vi "backup_strain_test_v4.vi"() -> ()   [LabVIEW 2014]
uses:
  <vilib>/LabVIEW Targets/FPGA/cRIO/shared/nicrio_ModuleControls/nicrio_cRIO-9237_DataRatesRing.ctl
  <vilib>/LabVIEW Targets/FPGA/cRIO/shared/nicrio_ModuleControls/nicrio_cRIO-9237_ExcitationVoltageRing.ctl
  <vilib>/rvi/Emulation/niFpgaGetClockAttributes.vi
  <vilib>/rvi/Emulation/niFpgaSctlEmulationGetInTimedLoop.vi
  <vilib>/rvi/Emulation/niFpgaEmulationReportErrorSimple.vi
  <vilib>/rvi/Emulation/niFpgaProcessEmulError.vi
  <vilib>/rvi/interface/RandomDataEmulation/nirviRandomDataMultiElementFPGAFIFO.vi
  <instcachedir>/0/nirviRandomDataMultiElementFPGAFIFO_AD0CFC12EF974623A9C2E4184BC062B2.lvgen/nirviRandomDataMultiElementFPGAFIFO_AD0CFC12EF974623A9C2E4184BC062B2_023.vi
  <vilib>/rvi/interface/RandomDataEmulation/niFpgaRandomDataHandleErrors.vi
  <vilib>/rvi/Emulation/niFpgaCriticalErrorInLSC.vi
  <vilib>/rvi/eio/common/nirviEmuTemplatePropertySet_errors.vi
  <vilib>/rvi/eio/common/nirviEmuTemplateMethod_errors.vi
  <vilib>/rvi/DataTransferAndStorage/Container/XNode/niFpgaContainer.xnode
  <vilib>/rvi/interface/RandomDataEmulation/nirviRandomDataFpgaMultiElementTemplate.vi
  <vilib>/eio/EIOPropertyNode/EIOPropertyNode.xnode
  <vilib>/eio/EIONode/EIONode.xnode
  <vilib>/rvi/Analysis/measure/butterworth/XNode/niFpgaButterworthFilter.xnode
  <vilib>/rvi/eio/common/nirviEmuTemplatePropertyGet_errors.vi
  <vilib>/rvi/eio/common/nirviEmuTemplatePropertyGet_noerrors.vi
  <vilib>/rvi/eio/common/nirviEmuTemplatePropertySet_noerrors.vi
panel:
  out "Strain(mean)":fxp<+/-,32,4>
  out "Loop rate (kHz)":fxp<+/-,36,7>
  in  "Strain filter coeff.":i32[](array[numeric])=[-850883994, 1909449570, 3794062, -975456236, 2033039520, 4039635]
  out "Force":fxp<+/-,32,10>
  out "Strain":fxp<+/-,42,8>
  out "Fileterd data":fxp<+/-,32,4>
  out "Raw Force":fxp<+/-,32,10>
  in  "S/F coeff":fxp<+/-,41,4>
  out "Raw Strain":fxp<+/-,42,8>
  in  "Reset":bool
  in  "Stop":bool
  out "Mod6/AI2":fxp<+/-,32,4>
  in  "Shunt Cal Enable":bool
  in  "Half-Bridge Enable":bool
  in  "Excitation Voltage":T1 items=["2.5 Volts", "3.3 Volts", "5.0 Volts", "10.0 Volts", "External Excitation"]
  in  "Data Rate":T2=1 items=["50.000 kS/s (NI 9237)"=1, "25.000 kS/s (NI 9237)"=2, "16.667 kS/s (NI 9237)"=3, "12.500 kS/s (NI 9237)"=4, "10.000 kS/s (NI 9237)"=5, "8.333 kS/s (NI 9237)"=6, "7.143 kS/s (NI 9237)"=7, "6.250 kS/s (NI 9237)"=8, "5.556 kS/s (NI 9237)"=9, "5.000 kS/s (NI 9237)"=10, "4.545 kS/s (NI 9237)"=11, "4.167 kS/s (NI 9237)"=12, "3.846 kS/s (NI 9237)"=13, "3.571 kS/s (NI 9237)"=14, "3.333 kS/s (NI 9237)"=15, "3.125 kS/s (NI 9237)"=16, "2.941 kS/s (NI 9237)"=17, "2.778 kS/s (NI 9237)"=18, "2.632 kS/s (NI 9237)"=19, "2.500 kS/s (NI 9237)"=20, "2.381 kS/s (NI 9237)"=21, "2.273 kS/s (NI 9237)"=22, "2.174 kS/s (NI 9237)"=23, "2.083 kS/s (NI 9237)"=24, "2.000 kS/s (NI 9237)"=25, "1.923 kS/s (NI 9237)"=26, "1.852 kS/s (NI 9237)"=27, "1.786 kS/s (NI 9237)"=28, "1.724 kS/s (NI 9237)"=29, "1.667 kS/s (NI 9237)"=30, "1.613 kS/s (NI 9237)"=31]
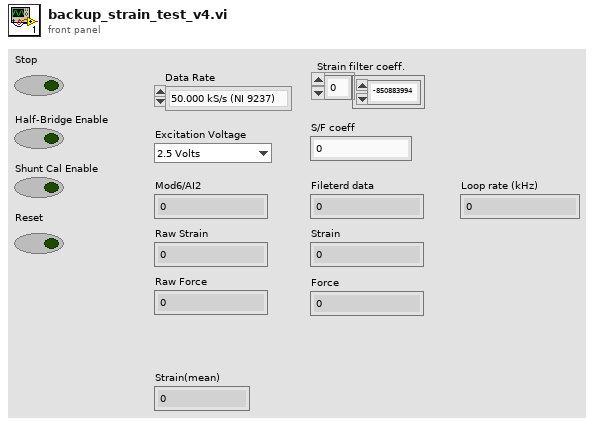
[diagram p1: front panel]
types:
  T1 = typedef "nicrio_cRIO-9237_ExcitationVoltageRing.ctl" = u8
  T2 = typedef "nicrio_cRIO-9237_DataRatesRing.ctl" = u8
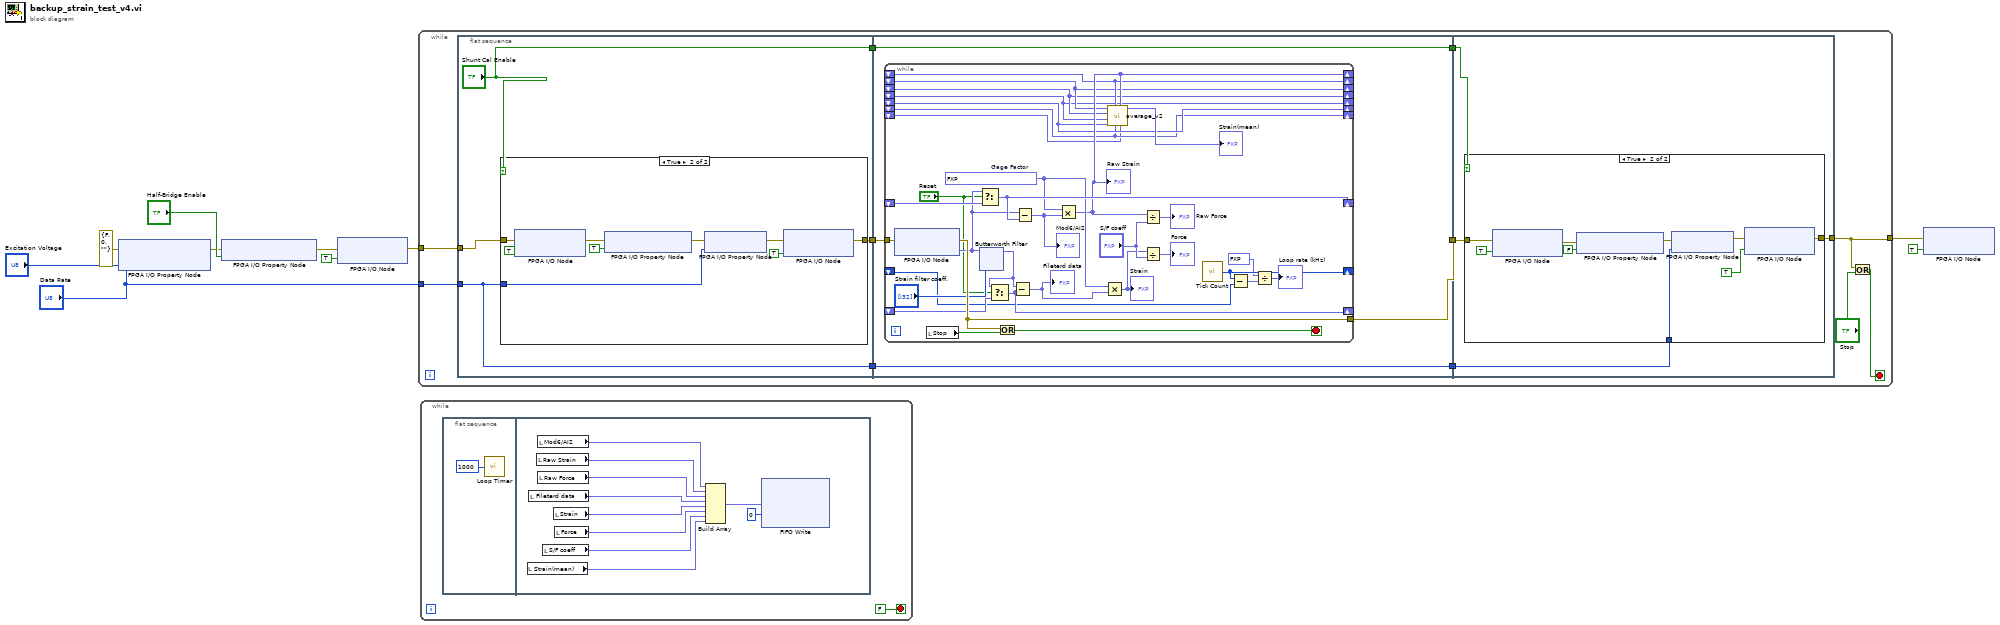
[diagram p0: block diagram]
diagram:
  n1 = xnode "FPGA I/O Property Node"("error in"=errorcluster {"status"=FALSE, "code"=0, "source"=""}, "Data Rate"="Data Rate", "Excitation Voltage"="Excitation Voltage") -> ("error out"=w7:errorcluster)  [unwired: 1 in, 1 out]
  n2 = xnode "FPGA I/O Property Node"("error in"=w7, "Half-Bridge Enable"="Half-Bridge Enable") -> ("error out"=w6:errorcluster)  [unwired: 1 in, 1 out]
  n3 = xnode "FPGA I/O Node"("error in"=w6, "Mod6/Start"=TRUE) -> ("error out"=w4:errorcluster)  [unwired: 1 in, 1 out]
  n4 = while {
    tunnel: w4 -> [w21]
    tunnel: "Data Rate" -> [w20]
    tunnel: [w12] -> w2
    stop <- w13 stop-if-true
    n5 = flat-sequence {
      tunnel: w21 -> [w25]
      tunnel: w20 -> [w24]
      tunnel: [w24] -> w19
      tunnel: ["Shunt Cal Enable"] -> w18
      tunnel: [w22] -> w17
      tunnel: w19 -> [w37]
      tunnel: w18 -> [w38]
      tunnel: w17 -> [w39]
      tunnel: [w38] -> w16
      tunnel: [w36] -> w15
      tunnel: [w37] -> w14
      tunnel: w16 -> [w84]
      tunnel: w15 -> [w83]
      tunnel: w14 -> [w82]
      tunnel: [w81] -> w12
      frame #0 {
        n6 = case shown="True" "Shunt Cal Enable" {
          tunnel: w25 -> [w26 w33]
          tunnel: w24 -> [_ w31]
          tunnel: [w26 w28] -> w22
          frame False {
          }
          frame True {
            n7 = xnode "FPGA I/O Node"("error in"=w33, "Mod6/Stop"=TRUE) -> ("error out"=w34:errorcluster)  [unwired: 1 in, 1 out]
            n8 = xnode "FPGA I/O Property Node"("error in"=w34, "Shunt Cal Enable"=TRUE) -> ("error out"=w32:errorcluster)  [unwired: 1 in, 1 out]
            n9 = xnode "FPGA I/O Property Node"("error in"=w32, "Data Rate"=w31) -> ("error out"=w30:errorcluster)  [unwired: 1 in, 1 out]
            n10 = xnode "FPGA I/O Node"("error in"=w30, "Mod6/Start"=TRUE) -> ("error out"=w28:errorcluster)  [unwired: 1 in, 1 out]
          }
        }
      }
      frame #1 {
        n11 = while {
          tunnel: w39 -> [w72]
          tunnel: [w70] -> w36
          shift-right: [w68] -> _
          shift-left: _ -> [w69]
          shift-right: [w64] -> _
          shift-left: _ -> [w65]
          shift-right: [w53] -> _
          shift-left: _ -> [w54]
          shift-right: [w48] -> _
          shift-left: _ -> [w46]
          shift-right: [w46] -> _
          shift-left: _ -> [w45]
          shift-right: [w45] -> _
          shift-left: _ -> [w44]
          shift-right: [w44] -> _
          shift-left: _ -> [w43]
          shift-right: [w43] -> _
          shift-left: _ -> [w42]
          shift-right: [w42] -> _
          shift-left: _ -> [w41]
          shift-right: [w41] -> _
          shift-left: _ -> [w40]
          stop <- w57 stop-if-true
          w62 = fxp<+,20,2> 2.115001678466797  # Gage Factor
          n12 = xnode "FPGA I/O Node"("error in"=w72) -> ("error out"=w70:errorcluster, "Mod6/AI2"=w66:fxp<+/-,24,-4>)  [unwired: 1 in, 1 out]
          n13 = local read "Stop"() -> (w71:bool)
          n14 = xnode "Butterworth Filter"("input data"=w66, "scaled coefficients"="Strain filter coeff.") -> ("output data"=w63:fxp<+/-,28,0>)  [unwired: 1 in]
          n15 = Select(t=w66, s="Reset", f=w69) -> (s? t:f=w68:fxp<+/-,24,-4>)
          n16 = Select(t=w63, s="Reset", f=w65) -> (s? t:f=w64:fxp<+/-,28,0>)
          n17 = Or(x=w70, y=w71) -> (x .or. y?=w57:bool)
          n18 = Subtract(x=w63, y=w64) -> (x-y=w61:fxp<+/-,32,16>)
          "Fileterd data" <- w61
          n19 = Subtract(x=w66, y=w68) -> (x-y=w67:fxp<+/-,25,-3>)
          "Mod6/AI2" <- w67
          n20 = Multiply(x=w62, y=w67) -> (x*y=w48:fxp<+/-,41,6>)
          "Raw Strain" <- w48
          n21 = Multiply(x=w62, y=w61) -> (x*y=w59:fxp<+/-,41,6>)
          "Strain" <- w59
          n22 = call "average_v2.vi"("Numeric 8"=w40, "Numeric"=w48, "Numeric 7"=w41, "Numeric 2"=w46, "Numeric 6"=w42, "Numeric 5"=w43, "Numeric 4"=w44, "Numeric 3"=w45) -> ("Mean (8pt)"=→"Strain(mean)":fxp<+/-,32,4>)  [unwired: 1 in, 2 out]
          n23 = Divide(x=w48, y="S/F coeff") -> (x/y=→"Raw Force":fxp<+/-,64,44>)
          n24 = Divide(x=w59, y="S/F coeff") -> (x/y=→"Force":fxp<+/-,64,44>)
          n25 = call "Tick Count"() -> ("Tick Count(uSec)"=w53:u32)
          n26 = Subtract(x=w53, y=w54) -> (x-y=w51:fxp<+/-,32,16>)
          n27 = Divide(x=fxp<+,7,10> 1000.0, y=w51) -> (x/y=→"Loop rate (kHz)":fxp<+/-,40,27>)
        }
      }
      frame #2 {
        n28 = case shown="True" w84 {
          tunnel: w83 -> [w85 w93]
          tunnel: w82 -> [_ w89]
          tunnel: [w85 w86] -> w81
          frame False {
          }
          frame True {
            n29 = xnode "FPGA I/O Node"("error in"=w93, "Mod6/Stop"=TRUE) -> ("error out"=w91:errorcluster)  [unwired: 1 in, 1 out]
            n30 = xnode "FPGA I/O Property Node"("error in"=w91, "Shunt Cal Enable"=FALSE) -> ("error out"=w90:errorcluster)  [unwired: 1 in, 1 out]
            n31 = xnode "FPGA I/O Property Node"("error in"=w90, "Data Rate"=w89) -> ("error out"=w88:errorcluster)  [unwired: 1 in, 1 out]
            n32 = xnode "FPGA I/O Node"("error in"=w88, "Mod6/Start"=TRUE) -> ("error out"=w86:errorcluster)  [unwired: 1 in, 1 out]
          }
        }
      }
    }
    n33 = Or(x=w12, y="Stop") -> (x .or. y?=w13:bool)
  }
  n34 = while {
    stop <- FALSE stop-if-true
    n35 = flat-sequence {
      frame #0 {
        n36 = call "Loop Timer"("Count(uSec)"=u32 1000) -> ()  [unwired: 1 out]
      }
      frame #1 {
        n37 = local read "Strain(mean)"() -> (w97:fxp<+/-,32,4>)
        n38 = local read "Fileterd data"() -> (w103:fxp<+/-,32,4>)
        n39 = local read "Raw Strain"() -> (w105:fxp<+/-,42,8>)
        n40 = local read "Mod6/AI2"() -> (w106:fxp<+/-,32,4>)
        n41 = local read "Raw Force"() -> (w104:fxp<+/-,32,10>)
        n42 = local read "S/F coeff"() -> (w100:fxp<+/-,41,4>)
        n43 = local read "Strain"() -> (w102:fxp<+/-,42,8>)
        n44 = local read "Force"() -> (w101:fxp<+/-,32,10>)
        n45 = Build Array(w106, w105, w104, w103, w102, w101, w100, w97) -> (w99:fxp<+/-,47,10>[])
        n46 = xnode ("FIFO Write")("Element"=w99, "Timeout"=0) -> ()  [unwired: 1 in, 2 out]
      }
    }
  }
  n47 = xnode "FPGA I/O Node"("error in"=w2, "Mod6/Stop"=TRUE) -> ()  [unwired: 1 in, 2 out]
